vi "Set Humidity.vi"(5 "Humidity":dbl=2.0 min=2.0 max=98.0 step=1.0, 6 "Lower Limit":dbl=nan, 7 "Upper Limit":dbl=nan, 8 "error in (no error)":errorcluster, 10 "Address (0)":i32, 11 "VISA resource name":refnum<visa-resource-name>) -> (0 "error out":errorcluster, 3 "VISA resource name out":refnum<visa-resource-name>)   [LabVIEW 2021, in "Environment Chamber.lvlib" / "Climatic Chamber.lvlib"]
doc: "<b>Humidity-related settings</B>\n\nChanges the humidity set point, upper limit alarm, lower limit alarm or all values together in constant mode No.1"
uses:
  Climatic Chamber.lvlib
panel:
  out "NACK":bool
  out "Error":bool
  out "ACK":bool
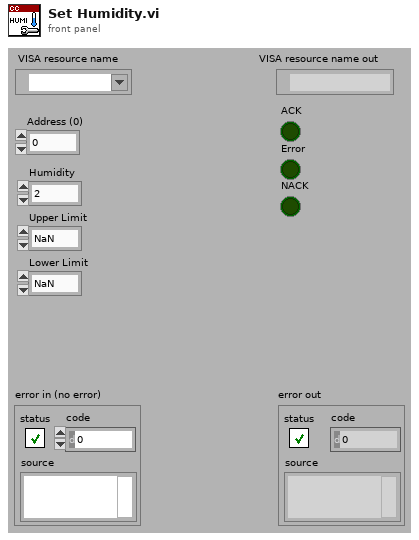
[diagram p1: front panel]
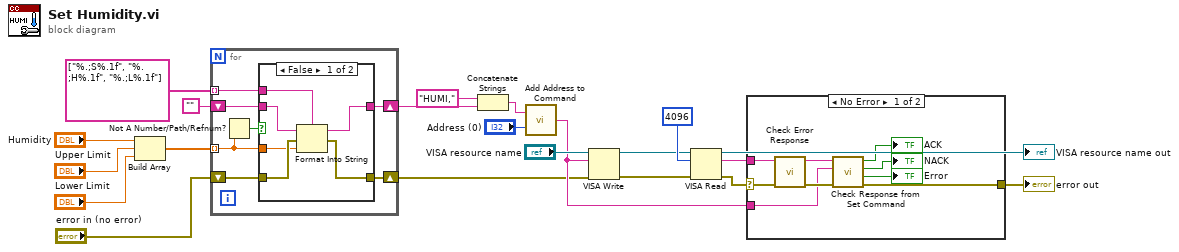
[diagram p0: block diagram]
diagram:
  n1 = Build Array("Humidity", "Upper Limit", "Lower Limit") -> (w6:dbl[])
  n2 = for {
    tunnel: w6 -> [w27] mode=indexing
    shift-right: [w26] -> w3
    shift-left: "" -> [w25]
    tunnel: string[] ["%.;S%.1f", "%.;H%.1f", "%.;L%.1f"] -> [w24] mode=indexing
    shift-right: [w22] -> w1
    shift-left: "error in (no error)" -> [w23]
    n3 = Not A Number/Path/Refnum?(number/path/refnum=w27) -> (NaN/Path/Refnum?=w28:bool)
    n4 = case shown="False" w28 {
      tunnel: w27 -> [w33 _]
      tunnel: [w31 w36] -> w26
      tunnel: w25 -> [w32 w36]
      tunnel: w24 -> [w30 _]
      tunnel: w23 -> [w34 w35]
      tunnel: [w29 w35] -> w22
      frame False {
        n5 = Format Into String(format string=w30, initial string=w32, error in=w34, w33) -> (resulting string=w31:string, error out=w29:errorcluster)
      }
      frame True {
      }
    }
  }
  n6 = Concatenate Strings("HUMI,", w3) -> (w10:string)
  n7 = call "Add Address to Command.vi"("Address (0)"="Address (0)", "Command"=w10) -> ("Command OUT"=w12:string)
  n8 = VISA Write(VISA resource name="VISA resource name", write buffer=w12, error in (no error)=w1) -> (VISA resource name out=w19:refnum<visa-resource-name>, error out=w18:errorcluster)  [unwired: 1 out]
  n9 = VISA Read(VISA resource name=w19, byte count=u32 4096, error in (no error)=w18) -> (VISA resource name out=→"VISA resource name out":refnum<visa-resource-name>, read buffer=w14:string, error out=w15:errorcluster)  [unwired: 1 out]
  n10 = case shown="No Error" w15 {
    selector: w15 -> [w44 w46]
    tunnel: w14 -> [w45 _]
    tunnel: [w40 w46] -> w13
    tunnel: w12 -> [w41 _]
    frame No Error {
      n11 = call "Check Error Response.vi"("error in (no error)"=w44, "read String"=w45) -> ("error out"=w43:errorcluster, "String out"=w42:string)  [unwired: 7 in, 1 out]
      n12 = call "Check Response from Set Command.vi"("error in (no error)"=w43, "Command"=w41, "Response"=w42) -> ("error out"=w40:errorcluster, "Error"=→"Error":bool, "NACK"=→"NACK":bool, "ACK"=→"ACK":bool)  [unwired: 5 in]
    }
    frame Error {
    }
  }
  "error out" <- w13
